vi "Execute SequenceFile.vi"() -> ()   [LabVIEW 2020]
uses:
  Engine/TS License Type.ctl
  Data Types/File Load Options.ctl
  VariableContainer/Set Value STR.vi
  VariableContainer/Set Value BOOL.vi
  VariableContainer/Set Value U64.vi
  Execution/Set Entry Sequence.vi
  Execution/Set Sequence File.vi
  Execution/Set Parameters.vi
  Execution/Execution.lvclass
  Engine/Engine.lvclass
  VariableContainer/VariableContainer.lvclass
  TSS.lvlib
  SequenceFile/SequenceFile.lvclass
  VariableContainer/Set Value VAR.vi
panel:
  out "Acquired License":T1
  in  "Terminate":bool
  in  "Resume":bool
  in  "Params":T2={"SerialNo"="ABC123", "TestBool"=TRUE, "DeviceID"=5648432}
  out "error out":errorcluster
  in  "Sequence":string="MainSequence"
  in  "SequenceFile Path":path=path "C:/dev/Negentropic/HTS/Test/Sequences/DisplaySerialNo.seq"
  # "The sequence will pause immediately when starting, choose resume to run it and get the dialog or terminate to cancel execution."
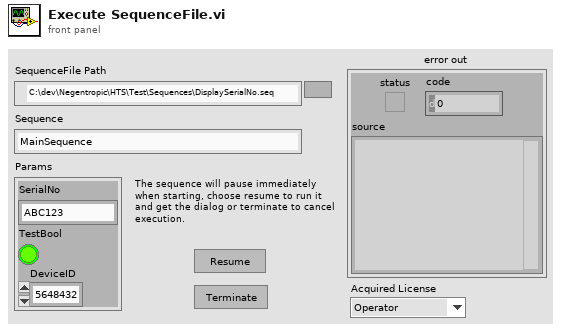
[diagram p1: front panel]
types:
  T1 = typedef "TSS.lvlib/Engine.lvclass/TS License Type.ctl" = enum16{"Operator", "CustomEditor", "SequenceEditor"}
  T2 = cluster{"SerialNo":string, "TestBool":bool, "DeviceID":u64}
  T3 = typedef "TSS.lvlib/File Load Options.ctl" = cluster{"Use Search Dirs? (T)":bool, "Conflict as Error? (T)":bool, "Check Station Model? (F)":bool, "Preload Modules? (T)":bool, "Skip Load Callback? (F)":bool, "Reload if Loaded? (F)":bool}
  T4 = typedef "TSS.lvlib/Engine.lvclass/Session Handle.ctl" = refnum<data-value>
  T5 = typedef "TSS.lvlib/Execution.lvclass/Session Handle.ctl" = refnum<data-value>
  T6 = typedef "TSS.lvlib/SequenceFile.lvclass/Session Handle.ctl" = refnum<data-value>
  T7 = typedef "TSS.lvlib/VariableContainer.lvclass/Session Handle.ctl" = refnum<data-value>
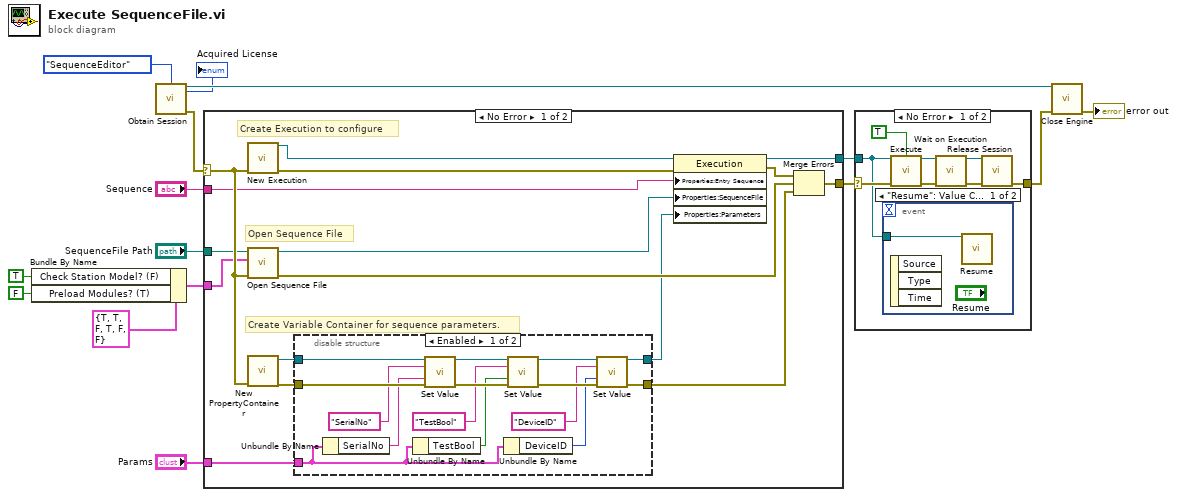
[diagram p0: block diagram]
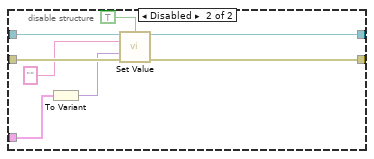
[diagram p2: hidden frame]
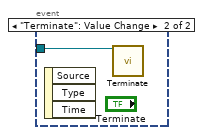
[diagram p4: hidden frame]
diagram:
  n1 = Bundle By Name(cluster=T3 {"Use Search Dirs? (T)"=TRUE, "Conflict as Error? (T)"=TRUE, "Check Station Model? (F)"=FALSE, "Preload Modules? (T)"=TRUE, "Skip Load Callback? (F)"=FALSE, "Reload if Loaded? (F)"=FALSE} ("Load Options"), "Check Station Model? (F)"=TRUE, "Preload Modules? (T)"=FALSE) -> (w11:T3)
  n2 = call "Obtain Session.vi"("TS License Type (Operator)"=TS_License_Type."SequenceEditor") -> ("Acquired License"=→"Acquired License":T1, "Session Handle"=w2:T4, "error out"=w10:errorcluster)  [unwired: 12 in]
  n3 = case shown="No Error" w10 {
    selector: w10 -> [w30 w55]
    tunnel: [w28 _] -> w8
    tunnel: "Sequence" -> [w23 _]
    tunnel: w11 -> [w18 _]
    tunnel: "SequenceFile Path" -> [w20 _]
    tunnel: [w26 w55] -> w9
    tunnel: "Params" -> [w25 _]
    frame No Error {
      # "Create Variable Container for sequence parameters."
      # "Open Sequence File"
      # "Create Execution to configure"
      n4 = call "New Execution.vi"("error in (no error)"=w30) -> ("Session Handle out"=w22:T5, "error out"=w21:errorcluster)  [unwired: 13 in]
      n5 = call "Open Sequence File.vi"("error in (no error)"=w30, "Load Options (Default)"=w18, "Path"=w20) -> ("error out"=w31:errorcluster, "Session Handle out"=w19:T6)  [unwired: 7 in]
      n6 = call "New PropertyContainer.vi"("error in (no error)"=w30) -> ("error out"=w16:errorcluster, "Session Handle out"=w17:T7)  [unwired: 9 in]
      n7 = disable-structure shown="Enabled" {
        disable-tunnel: [w46 w50] -> w29
        disable-tunnel: w16 -> [w45 w53]
        disable-tunnel: w17 -> [w37 w54]
        disable-tunnel: [w36 w49] -> w24
        disable-tunnel: w25 -> [w32 w51]
        frame Enabled {
          n8 = Unbundle By Name(w32) -> ("SerialNo"=w35:string)
          n9 = Unbundle By Name(w32) -> ("TestBool"=w34:bool)
          n10 = call-poly "Set Value.vi"("Session Handle in"=w37, "Lookup String"="SerialNo", "Value"=w35, "error in (no error)"=w45) -> ("Session Handle out"=w41:T7, "error out"=w43:errorcluster)  [unwired: 10 in]
          n11 = Unbundle By Name(w32) -> ("DeviceID"=w33:u64)
          n12 = call-poly "Set Value.vi"("Session Handle in"=w41, "Lookup String"="TestBool", "Value"=w34, "error in (no error)"=w43) -> ("Session Handle out"=w39:T7, "error out"=w44:errorcluster)  [unwired: 10 in]
          n13 = call-poly "Set Value.vi"("Session Handle in"=w39, "Lookup String"="DeviceID", "Value"=w33, "error in (no error)"=w44) -> ("Session Handle out"=w36:T7, "error out"=w46:errorcluster)  [unwired: 10 in]
        }
        frame Disabled {
          n14 = To Variant(anything=w51) -> (Variant=w48:variant)
          n15 = call-poly "Set Value.vi"("Session Handle in"=w54, "Skip Outer Cluster (T)"=TRUE, "Lookup String"="", "Value"=w48, "error in (no error)"=w53) -> ("Session Handle out"=w49:T7, "error out"=w50:errorcluster)  [unwired: 9 in]
        }
      }
      n16 = property class="Execution"(reference=w22, error in=w21, "Properties:Entry Sequence"=w23, "Properties:SequenceFile"=w19, "Properties:Parameters"=w24) -> (reference out=w28:T5, error out=w27:errorcluster)
      n17 = Merge Errors(w27, w31, w29) -> (w26:errorcluster)
    }
    frame Error {
    }
  }
  n18 = case shown="No Error" w9 {
    selector: w9 -> [w63 w66]
    tunnel: w8 -> [w62 _]
    tunnel: [w57 w66] -> w4
    frame No Error {
      n19 = event shown="[0] \"Resume\": Value Change" {
        selector: _ -> [_ _]
        dyn-events: _ -> [_ _]
        timeout: _ -> [_ _]
        tunnel: w62 -> [w64 w65]
        event "Resume": Value Change {
          n20 = event-data() -> ()  [unwired: 1 in, 3 out]
          n21 = call "Resume.vi"("Session Handle in"=w64) -> ()  [unwired: 13 in, 2 out]
        }
        event "Terminate": Value Change {
          n22 = event-data() -> ()  [unwired: 1 in, 3 out]
          n23 = call "Terminate.vi"("Session Handle in"=w65) -> ()  [unwired: 13 in, 2 out]
        }
      }
      n24 = call "Execute.vi"("Session Handle in"=w62, "Break at First Step? (F)"=TRUE, "error in (no error)"=w63) -> ("Session Handle out"=w59:T5, "error out"=w60:errorcluster)  [unwired: 11 in]
      n25 = call "Wait on Execution.vi"("Session Handle in"=w59, "error in (no error)"=w60) -> ("Session Handle out"=w56:T5, "error out"=w58:errorcluster)  [unwired: 11 in, 1 out]
      n26 = call "Release Session.vi"("Session Handle"=w56, "error in (no error)"=w58) -> ("error out"=w57:errorcluster)  [unwired: 13 in]
    }
    frame Error {
    }
  }
  n27 = call "Close Engine.vi"("Session Handle in"=w2, "error in (no error)"=w4) -> ("error out"=→"error out":errorcluster)  [unwired: 13 in]
